vi "RD SDK VERSION.vi"(8 "error in (no error)":errorcluster caption="错误输入（无错误）") -> (0 "error out":errorcluster caption="错误输出", 2 "Description out":string, 3 "function return":i32)   [LabVIEW 2018, in "InstrumentsPlayground.lvlib"]
doc: "CLIFFAPI int CliffEnumDeviceInfo (int i, char* Description,char* SerialNumber,FT_HANDLE *handle);"
uses:
  InstrumentsPlayground.lvlib
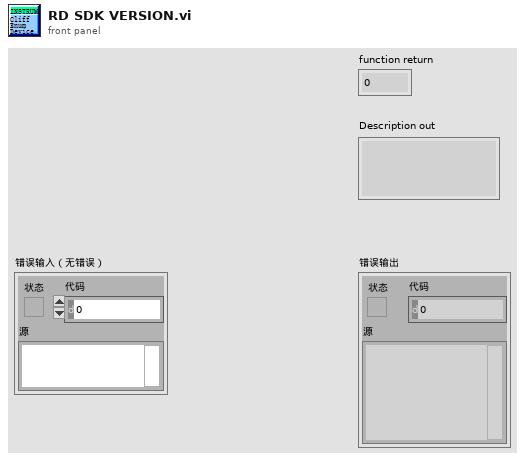
[diagram p1: front panel]
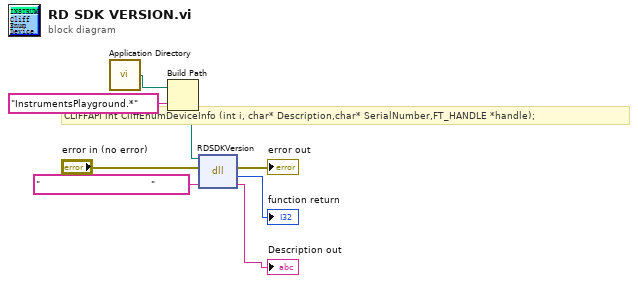
[diagram p0: block diagram]
diagram:
  # "CLIFFAPI int CliffEnumDeviceInfo (int i, char* Description,char* SerialNumber,FT_HANDLE *handle);"
  n1 = call <vilib>:"Application Directory.vi"() -> ("Application Directory"=w4:path)
  n2 = Build Path(base path=w4, name or relative path="InstrumentsPlayground.*" ("名称或相对路径")) -> (appended path=w3:path)
  n3 = dll-call lib="E:/work/YZCourse_Xtext/Cliff/API/IPLabView lib/InstrumentsPlayground.dll" fn="RDSDKVersion"(path in=w3, error in="error in (no error)", "version"="                                     ") -> (error out=→"error out":errorcluster, "返回类型"=→"function return":i32, "version"=→"Description out":string)  [unwired: 1 in, 1 out]
